vi "createQueues.vi"(8 "error in (no error)":errorcluster, 11 "tcpServerBase in":refnum<class "TcpServerBase.lvclass">) -> (0 "error out":errorcluster, 3 "tcpServerBase out":refnum<class "TcpServerBase.lvclass">)   [LabVIEW 2018, in "TcpServerBase.lvclass"]
doc: "Create server queue and client queue to communicate differents loops in LabVIEW TCP Server."
uses:
  TcpServerBase.lvclass
  TcpServerBase.lvclass/TcpServerBase.ctl
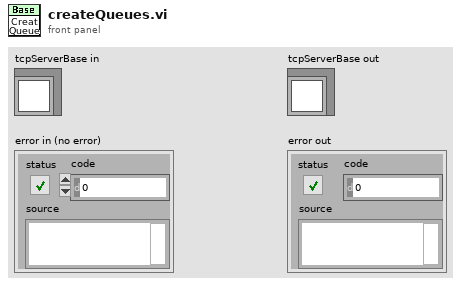
[diagram p1: front panel]
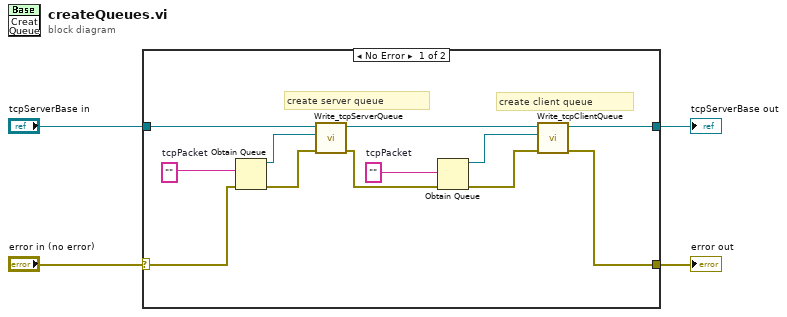
[diagram p0: block diagram]
diagram:
  n1 = case shown="No Error" "error in (no error)" {
    selector: "error in (no error)" -> [w13 w18]
    tunnel: "tcpServerBase in" -> [w16 w17]
    tunnel: [w14 w17] -> w3
    tunnel: [w9 w18] -> w1
    frame No Error {
      w6 = ""  # tcpPacket
      w7 = ""  # tcpPacket
      # "create client queue"
      # "create server queue"
      n2 = Obtain Queue(element data type=w7, error in (no error)=w13) -> (queue out=w5:refnum<queue>, error out=w12:errorcluster)  [unwired: 3 in, 1 out]
      n3 = call "Write_tcpServerQueue.vi"("error in (no error)"=w12, "tcpServerQueue"=w5, "TcpServerBase in"=w16) -> ("error out"=w11:errorcluster, "TcpServerBase out"=w15:refnum<class "TcpServerBase.lvclass">)  [unwired: 7 in]
      n4 = Obtain Queue(element data type=w6, error in (no error)=w11) -> (queue out=w8:refnum<queue>, error out=w10:errorcluster)  [unwired: 3 in, 1 out]
      n5 = call "Write_tcpClientQueue.vi"("error in (no error)"=w10, "tcpClientQueue"=w8, "TcpServerBase in"=w15) -> ("error out"=w9:errorcluster, "TcpServerBase out"=w14:refnum<class "TcpServerBase.lvclass">)  [unwired: 7 in]
    }
    frame Error {
    }
  }
  "error out" <- w1
  "tcpServerBase out" <- w3
